vi "Set End Effector Transform.vi"(8 "error in (no error)":errorcluster, 10 "end effector transform":T1, 11 "serial arm in":refnum<class "NI_Robotics_Serial Robot Arm.lvclass">) -> (0 "error out":errorcluster, 3 "serial arm out":refnum<class "NI_Robotics_Serial Robot Arm.lvclass">)   [LabVIEW 2017, in "NI_Robotics_Serial Robot Arm.lvclass"]
doc: "Sets the position of the end effector of a robotic arm."
uses:
  <vilib>/robotics/Kinematics/Robot/NI_Robotics_Serial Robot Arm.lvclass
  <vilib>/Analysis/Matrix/Datatypes/RealMatrix.ctl
  <vilib>/robotics/Kinematics/Robot/NI_Robotics_Serial Robot Arm.lvclass/NI_Robotics_Serial Robot Arm.ctl
  <vilib>/Analysis/Matrix/NI_Matrix.lvlib
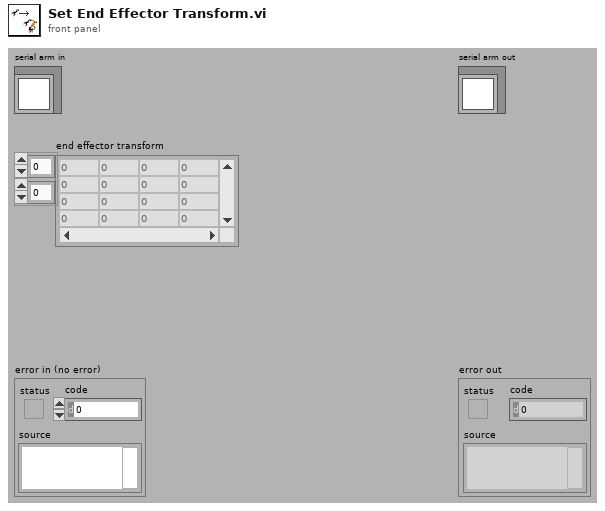
[diagram p1: front panel]
types:
  T1 = typedef "NI_Matrix.lvlib/RealMatrix.ctl" = dbl[][]
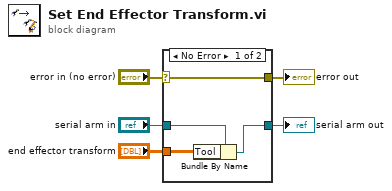
[diagram p0: block diagram]
diagram:
  n1 = case shown="No Error" "error in (no error)" {
    selector: "error in (no error)" -> [w9 w10]
    tunnel: [w9 w10] -> w4
    tunnel: [w7 w11] -> w2
    tunnel: "serial arm in" -> [w8 w11]
    tunnel: "end effector transform" -> [w6 _]
    frame No Error {
      n2 = Bundle By Name(cluster=w8, "Tool"=w6) -> (w7:refnum<class "NI_Robotics_Serial Robot Arm.lvclass">)
    }
    frame Error {
    }
  }
  "error out" <- w4
  "serial arm out" <- w2
